vi "Calc Roll.vi"(10 "Position":dbl) -> (2 "Roll":dbl)   [LabVIEW 2014]
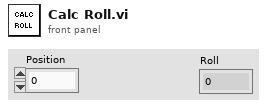
[diagram p1: front panel]
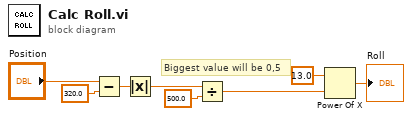
[diagram p0: block diagram]
diagram:
  # "Biggest value will be 0,5"
  n1 = Subtract(x="Position", y=320.0) -> (x-y=w6:dbl)
  n2 = Absolute Value(x=w6) -> (abs(x)=w5:dbl)
  n3 = Divide(x=w5, y=500.0) -> (x/y=w2:dbl)
  n4 = Power Of X(1:w2, 2:13.0 ("y")) -> (0:→"Roll":dbl)
